vi "Frame create.vi"(7 "Command":string, 8 "error in (no error)":errorcluster, 11 "ISO 15693 DOWN in":refnum<class "ISO 15693 DOWN.lvclass">) -> (0 "error out":errorcluster, 3 "ISO 15693 DOWN out":refnum<class "ISO 15693 DOWN.lvclass">)   [LabVIEW 2019, in "ISO 15693 DOWN.lvclass"]
uses:
  ISO 15693 DOWN.lvclass
  TypeDef/Store.ctl
  ISO 15693 DOWN.lvclass/ISO 15693 DOWN.ctl
  RFID system.lvclass
panel:
  in  "Value":u8[](array[numeric])=[227] format="%x"
  in  "Mask lenght":u8[](array[numeric])=[80] format="%x"
  in  "AFI":u8[](array[numeric])=[38] format="%x"
  in  "Inventory":u8[](array[numeric])=[31] format="%x"
  in  "Flag":u8[](array[numeric])=[49] format="%x"
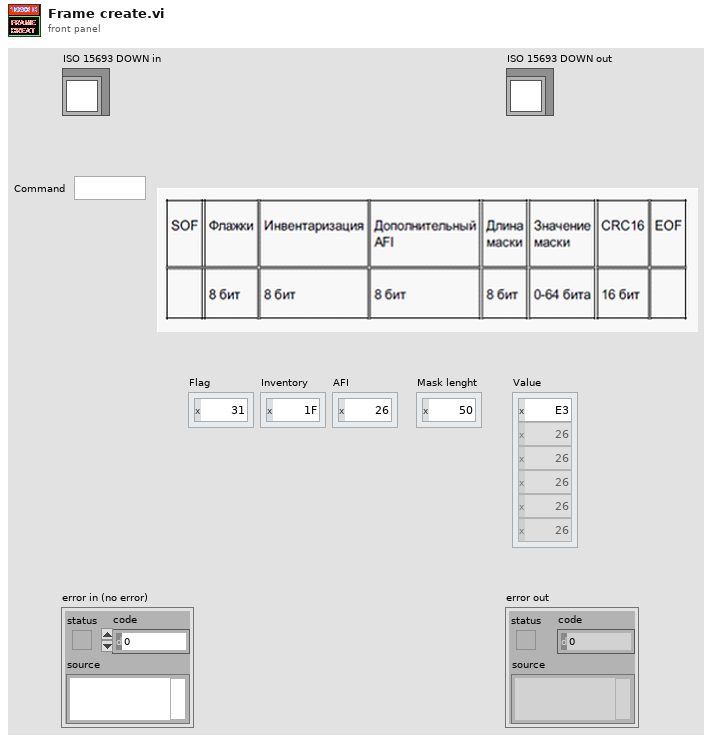
[diagram p1: front panel]
types:
  T1 = typedef "Store.ctl" = enum16{"envelope", "noise", "demSubCar", "CH_frame", "Decode", "demodulate", "in", "out", "sum", "subCarrier", "frame", "command", "encode", "modulate", "encode_UP", "modulate_up", "demod_up", "envelop_up", "sum_up", "out_up", "in_up"}
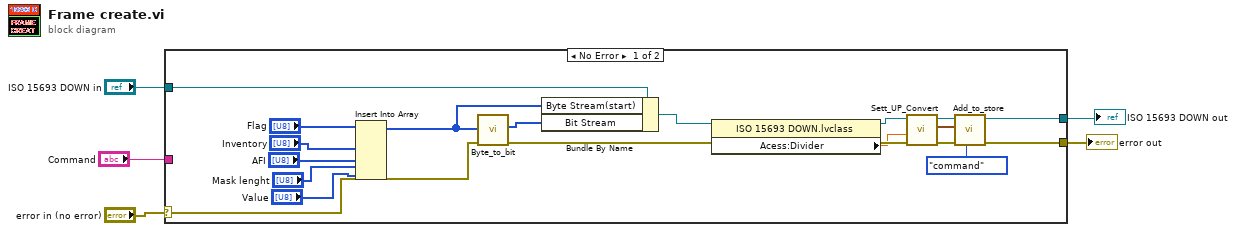
[diagram p0: block diagram]
diagram:
  n1 = case shown="No Error" "error in (no error)" {
    selector: "error in (no error)" -> [w19 w26]
    tunnel: [w12 w26] -> w4
    tunnel: "ISO 15693 DOWN in" -> [w18 w25]
    tunnel: [w13 w25] -> w2
    tunnel: "Command" -> [_ _]
    frame No Error {
      n2 = Insert Into Array(array="Flag", new element #1="Inventory", new element #2="AFI", new element #3="Mask lenght", new element #4="Value") -> (w6:u8[])  [unwired: 1 in]
      n3 = call "Byte_to_bit.vi"("Error In"=w19, "Array of byte"=w6) -> ("Error Out"=w10:errorcluster, "Arrray of bit"=w11:u8[])  [unwired: 5 in, 1 out]
      n4 = Bundle By Name(cluster=w18, "Byte Stream(start)"=w6, "Bit Stream"=w11) -> (w17:refnum<class "ISO 15693 DOWN.lvclass">)
      n5 = property class="ISO 15693 DOWN.lvclass"(reference=w17) -> (reference out=w8:refnum<class "ISO 15693 DOWN.lvclass">, "Acess:Divider"=w7:dbl)  [unwired: 1 in, 1 out]
      n6 = call-dynamic "Sett_UP_Convert.vi"("error in (no error)"=w10, "Divider(1)"=w7, "ISO 15693 DOWN in"=w8) -> ("error out"=w14:errorcluster, "Waveform"=w15:waveform(dbl), "ISO 15693 DOWN out"=w16:refnum<class "ISO 15693 DOWN.lvclass">)  [unwired: 6 in]
      n7 = call "Add_to_store.vi"("Store"=Store."command", "error in (no error)"=w14, "Waveform"=w15, "RFID system in"=w16) -> ("error out"=w12:errorcluster, "RFID system out"=w13:refnum<class "ISO 15693 DOWN.lvclass">)  [unwired: 6 in]
    }
    frame Error {
    }
  }
  "error out" <- w4
  "ISO 15693 DOWN out" <- w2
